vi "Get Valve Status.vi"(8 "error in (no error)":errorcluster, 11 "Aalborg GFC17 in":refnum<class "Aalborg GFC17.lvclass">) -> (0 "error out":errorcluster, 2 "Valve Status":T1, 3 "Aalborg GFC17 out":refnum<class "Aalborg GFC17.lvclass">)   [LabVIEW 2011, in "Aalborg GFC17.lvclass"]
uses:
  Aalborg GFC17.lvclass
  Mass Flow Controller/Valve Status.ctl
  Aalborg GFC17.lvclass/Aalborg GFC17.ctl
  <vilib>/DAQmx/read.llb/DAQmx Read (Analog DBL 1Chan 1Samp).vi
  <vilib>/DAQmx/miscellaneous.llb/DAQmx Fill In Error Info.vi
  Mass Flow Controller/Mass Flow Controller.lvclass
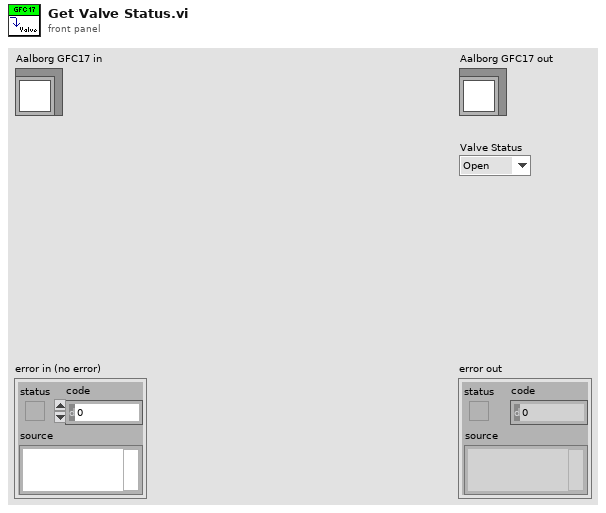
[diagram p1: front panel]
types:
  T1 = typedef "Mass Flow Controller.lvclass/Valve Status.ctl" = enum16{"Open", "Closed"}
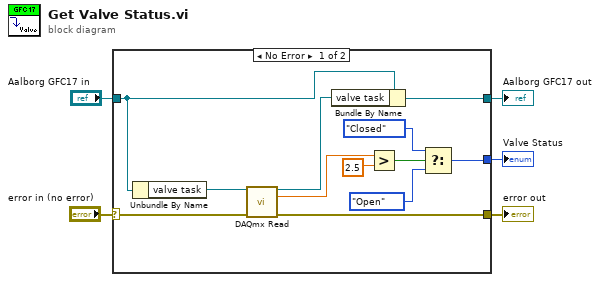
[diagram p0: block diagram]
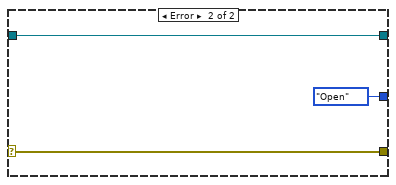
[diagram p2: hidden frame]
diagram:
  n1 = case shown="No Error" "error in (no error)" {
    selector: "error in (no error)" -> [w17 w20]
    tunnel: [w14 w20] -> w4
    tunnel: [w15 w19] -> w2
    tunnel: "Aalborg GFC17 in" -> [w16 w19]
    tunnel: [w7 Valve_Status."Open" ("Valve Status")] -> w1
    frame No Error {
      n2 = Unbundle By Name(w16) -> ("valve task"=w6:refnum<k21>)
      n3 = call-poly <vilib>:"DAQmx Read.vi"("task/channels in"=w6, "error in"=w17) -> ("task out"=w8:refnum<k21>, "data"=w13:dbl, "error out"=w14:errorcluster)  [unwired: 11 in]
      n4 = Bundle By Name(cluster=w16, "valve task"=w8) -> (w15:refnum<class "Aalborg GFC17.lvclass">)
      n5 = Greater?(x=w13, y=2.5) -> (0:w11:bool)
      n6 = Select(t=Valve_Status."Closed" ("Valve Status"), s=w11, f=Valve_Status."Open" ("Valve Status")) -> (s? t:f=w7:T1)
    }
    frame Error {
    }
  }
  "error out" <- w4
  "Aalborg GFC17 out" <- w2
  "Valve Status" <- w1
